vi "Command Reply.vi"(8 "Error In":errorcluster, 9 "Error?":bool, 10 "String":string, 11 "Network Info":T1 {"Last Comm Time" format="%<%H:%M:%S%3u\n%Y/%m/%d>T"; "Remote Port" format="%.0x"}) -> (0 "error out":errorcluster, 3 "TCP Network Connection out":refnum<k5>)   [LabVIEW 2023]
doc: "Author: Scott Hannahs <sth@magnet.fsu.edu>\nCopyright 2018 Florida State University, All rights reserved."
uses:
  RT Controls/Network Info.ctl
  RT Controls/RT System Auth Level.ctl
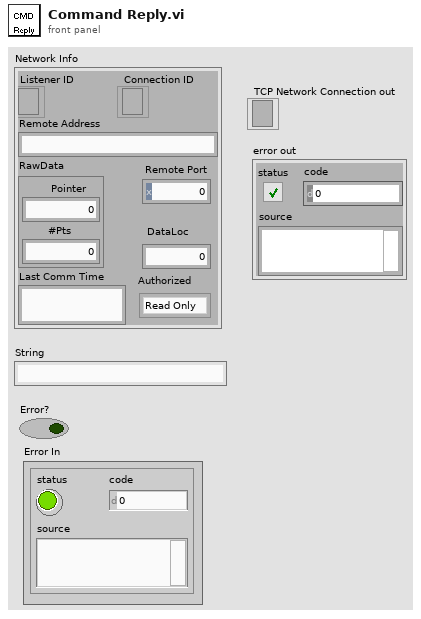
[diagram p1: front panel]
types:
  T1 = typedef "Network Info.ctl" = cluster{"Listener ID":refnum<k5>, "Connection ID":refnum<k5>, "Remote Address":string, "Remote Port":u16, "DataLoc":u32, "RawData":cluster{"#Pts":u32, "Pointer":u32}, "Last Comm Time":timestamp, "Authorized":T2}
  T2 = typedef "RT System Auth Level.ctl" = enum16{"Read Only", "Operator", "Admin"}
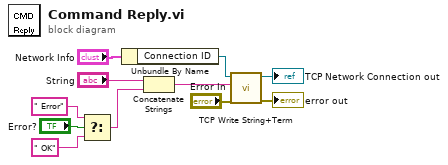
[diagram p0: block diagram]
diagram:
  n1 = Select(t=" Error" ("string"), s="Error?", f=" OK") -> (s? t:f=w7:string)
  n2 = Unbundle By Name("Network Info") -> ("Connection ID"=w3:refnum<k5>)
  n3 = Concatenate Strings("String", w7) -> (w5:string)
  n4 = call "TCP Write String+Term.vi"("Error In"="Error In", "Data"=w5, "connection ID"=w3) -> ("Error Out"=→"error out":errorcluster, "connection ID out"=→"TCP Network Connection out":refnum<k5>)  [unwired: 7 in]
